vi "Create.vi"() -> (0 "error out":errorcluster, 2 "Event":refnum<data-value>)   [LabVIEW 2021, in "jettl.lvlib"]
uses:
  jettl.lvlib
  Actor/Msg/Msg.lvclass
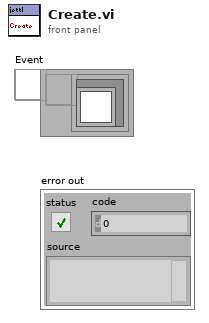
[diagram p1: front panel]
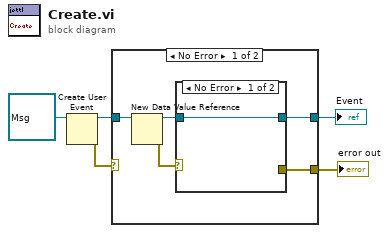
[diagram p0: block diagram]
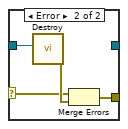
[diagram p2: hidden frame]
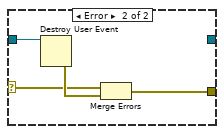
[diagram p3: hidden frame]
diagram:
  n1 = Create User Event(user event datatype=refnum<class "Msg.lvclass"> refnum ("Msg.lvclass")) -> (user event=w3:refnum<user-event>, error out=w2:errorcluster)  [unwired: 1 in]
  n2 = case shown="No Error" w2 {
    selector: w2 -> [_ w16]
    tunnel: w3 -> [w10 w19]
    tunnel: [w7 _] -> w1
    tunnel: [w8 w18] -> w5
    frame No Error {
      n3 = New Data Value Reference(data value=w10) -> (data value reference=w6:refnum<data-value>, error out=w9:errorcluster)  [unwired: 1 in]
      n4 = case shown="No Error" w9 {
        selector: w9 -> [_ w12]
        tunnel: [_ w15] -> w8
        tunnel: [w11 _] -> w7
        tunnel: w6 -> [w11 w14]
        frame No Error {
        }
        frame Error {
          n5 = call "Destroy.vi"("Event"=w14) -> ("error out"=w13:errorcluster)  [unwired: 10 in]
          n6 = Merge Errors(w12, w13) -> (w15:errorcluster)
        }
      }
    }
    frame Error {
      n7 = Destroy User Event(user event=w19) -> (error out=w17:errorcluster)  [unwired: 1 in]
      n8 = Merge Errors(w16, w17) -> (w18:errorcluster)
    }
  }
  "error out" <- w5
  "Event" <- w1
